vi "ByViServerInterfaceTemplate_CreateClass.vi"(1 "ProjectTreePosition(String or Project Item Ref)":variant, 2 "CreateClassData":T1, 3 "ClassTemplateFolder":path, 5 "error in (no error)":errorcluster, 6 "KeepLvClassRefOpen(False)":bool, 7 "HeaderToApply (take from VIRef or /use 2D-8bit header, Ignored if not wired)":variant) -> (15 "LVClassLibraryRefnum":refnum<vi>, 16 "TemplateVersionUsed":string, 19 "error out":errorcluster)   [LabVIEW 2020]
uses:
  <resource>/Framework/Providers/Open_GDS/ClassProviders/Provider_BaseClassInterface/CreateClassData.ctl
  <resource>/Framework/Providers/Open_GDS/ClassProviders/Common/LvClass_class/GDSLvCLass_ClassSettingsType.ctl
  <resource>/Framework/Providers/Open_GDS/ClassProviders/Common/LvClass_class/GDSLvClass_PlugIn.ctl
  <resource>/Framework/Providers/Open_GDS/ClassProviders/Common/LvClass_class/GDSLvClass_PlugInTypes.ctl
  <resource>/Framework/Providers/Open_GDS/ClassProviders/Provider_BaseClassInterface/ClassWriter_class/ClassWriter.lvclass
  <resource>/Framework/Providers/Open_GDS/ClassProviders/Provider_EndevoGOOP400/ClassWriterGOOP400_class/ClassWriterGOOP400.lvclass
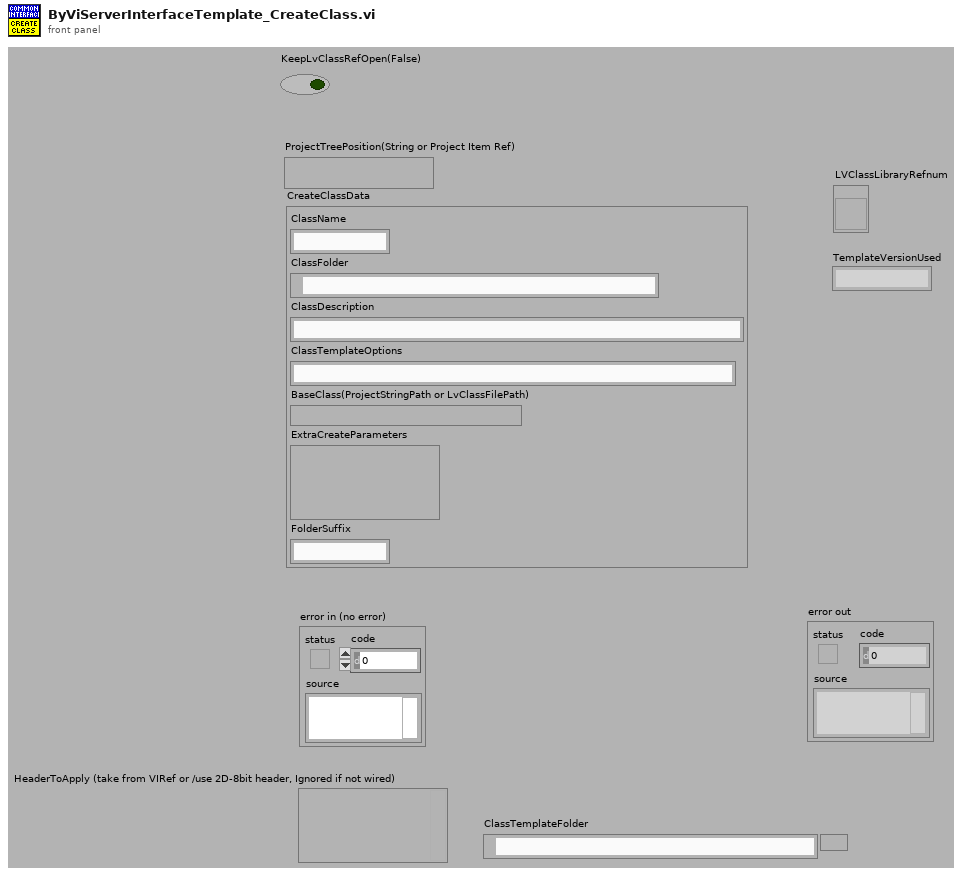
[diagram p1: front panel]
types:
  T1 = typedef "ClassWriter.lvclass/CreateClassData.ctl" = cluster{"ClassName":string, "ClassFolder":path, "ClassDescription":string, "ClassTemplateOptions":string, "BaseClass(ProjectStringPath or LvClassFilePath)":variant, "ExtraCreateParameters":variant, "FolderSuffix":string}
  T2 = cluster{"SubClass":bool, "ClassTemplateFiles":path[], "ClassName":string, "ClassFolder":path, "VIs":refnum<vi>[], "TemplateFolder":path, "ViSubDirs":string[], "TemplateName":string, "BaseClassFolder":path, "RootBaseClassFolder":path, "LvClassPath":path, "ClassRefnum":refnum<vi>, "ProjectRefnum":refnum<vi>, "LvClassFolderPath":path, "BaseClassName":string, "ClassItems":refnum<vi>[], "ViLocked":bool[], "ProjectItemOwner":refnum<vi>, "DeleteFiles":path[], "VIsBefore":refnum<vi>[], "BaseClassPath":path, "BaseConstructorBase":path, "TemplBaseConstructorBase":path, "TemplatePath":path, "TemplateVersion":string, "TemplateParentClass":refnum<vi>, "App":refnum<vi>, "Parent Class":refnum<vi>, "ParentVIs":refnum<vi>[], "TempClass":refnum<vi>}
  T3 = typedef "GDSLvCLass_ClassSettingsType.ctl" = cluster{"ClassProviderName":string, "ClassTemplateUsed":string, "ClassTemplateVersion":string, "ClassDescription":string, "PlugIns":T4[], "ConnectorPanePattern":string}
  T4 = typedef "GDSLvClass_PlugIn.ctl" = cluster{"Type":T5, "ID":string, "Version":string, "Path":path, "Name":string, "Data":variant}
  T5 = typedef "GDSLvClass_PlugInTypes.ctl" = enum16{"DesignPattern", "MethodTypes"}
  T6 = enum32{"invalid lock state", "Not Locked", "Locked (No Password)", "Password-protected"}
  T7 = typedef "Scripting_ConnectorPanePatternType.ctl" = u16
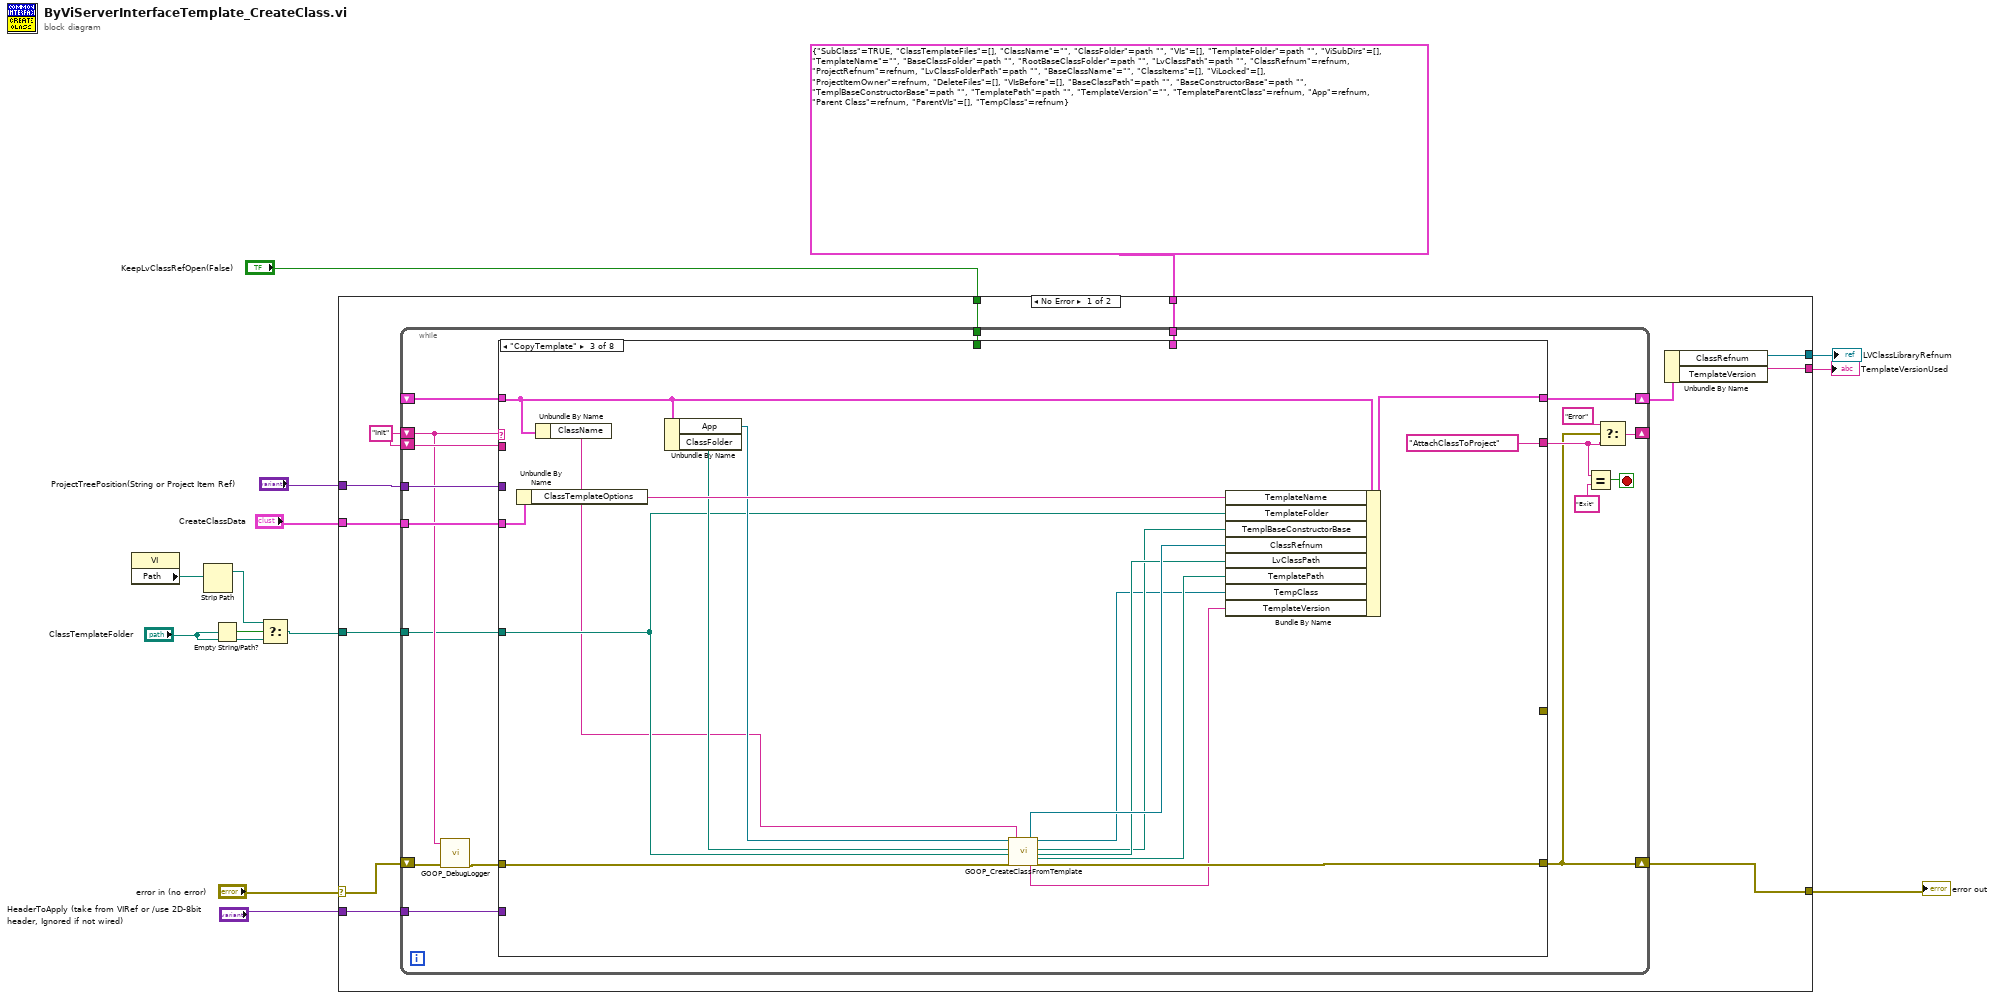
[diagram p0: block diagram]
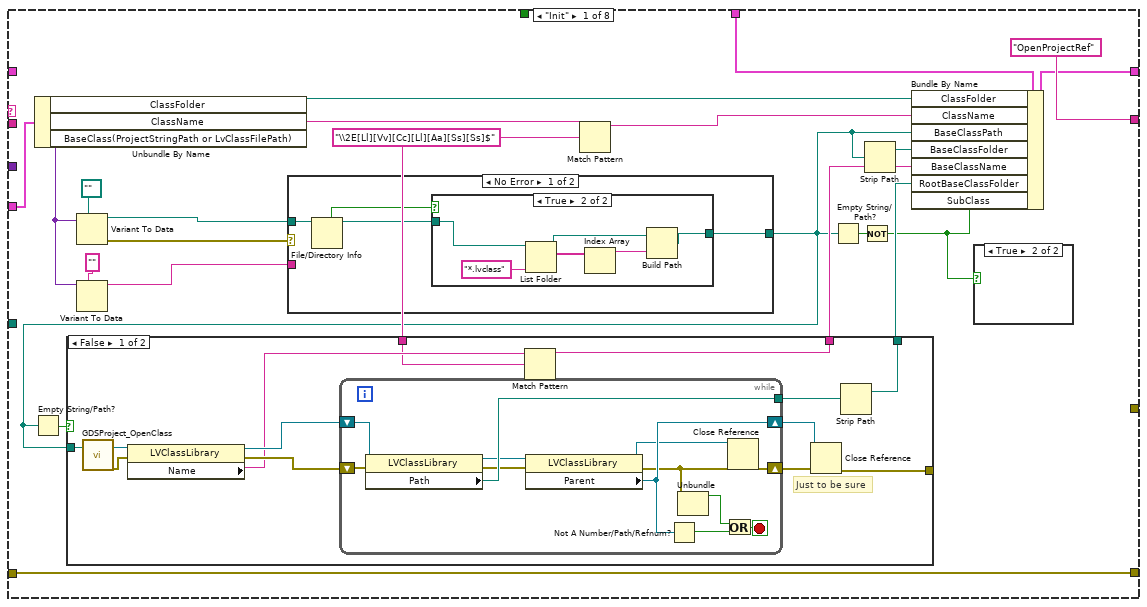
[diagram p2: hidden frame]
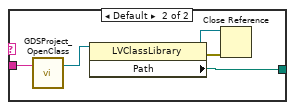
[diagram p7: hidden frame]
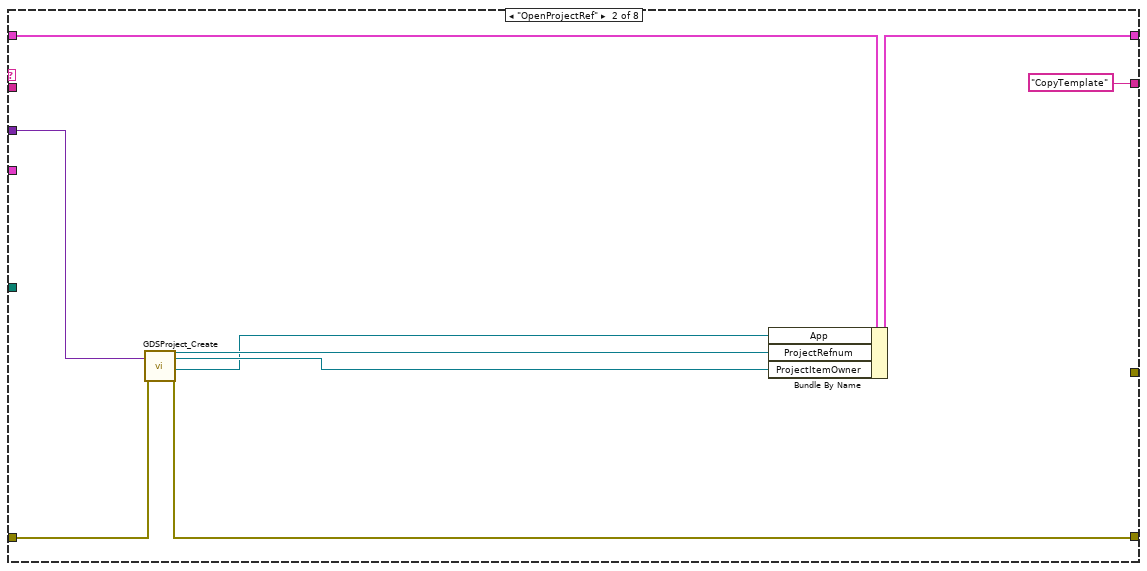
[diagram p8: hidden frame]
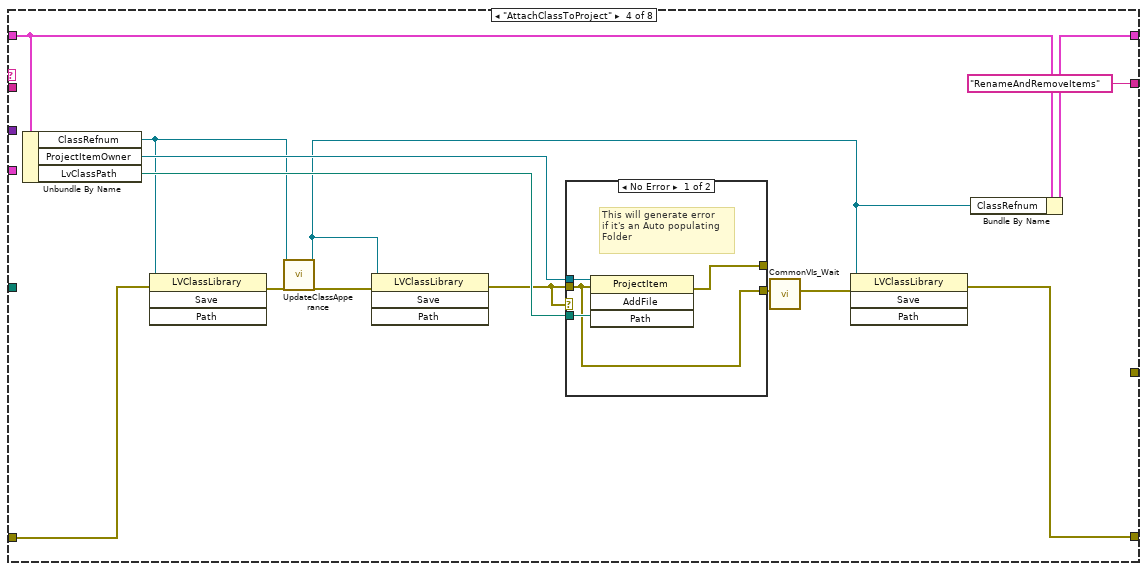
[diagram p9: hidden frame]
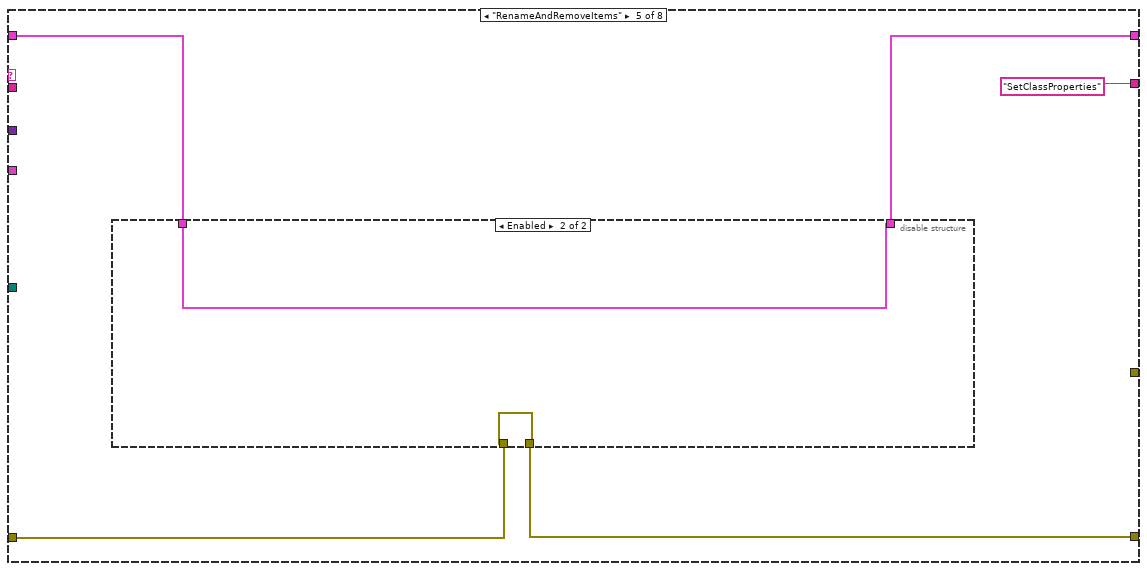
[diagram p11: hidden frame]
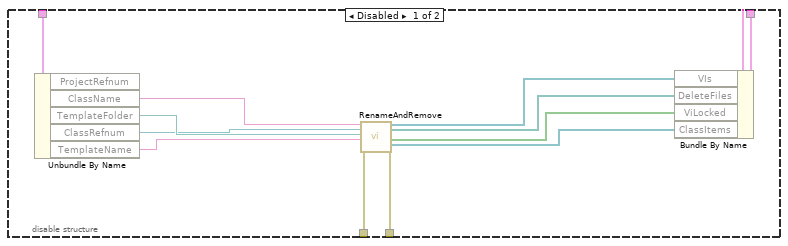
[diagram p12: hidden frame]
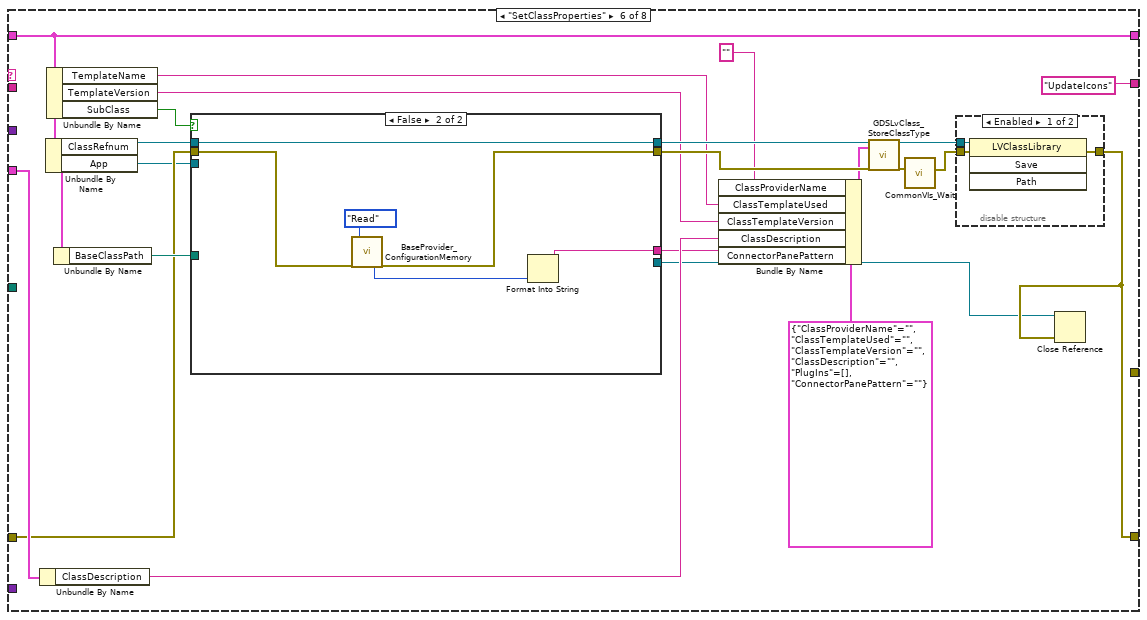
[diagram p13: hidden frame]
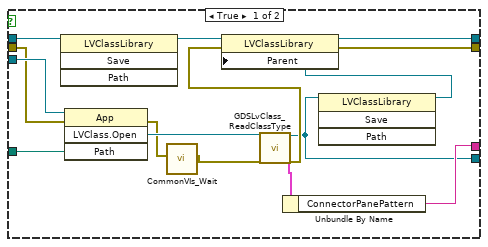
[diagram p15: hidden frame]
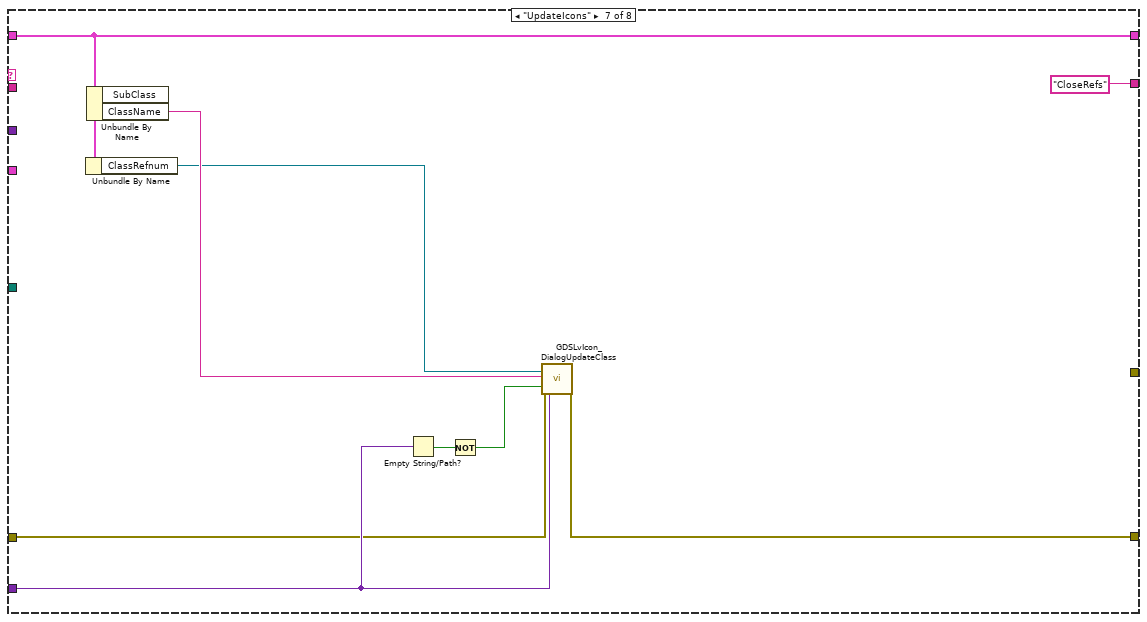
[diagram p16: hidden frame]
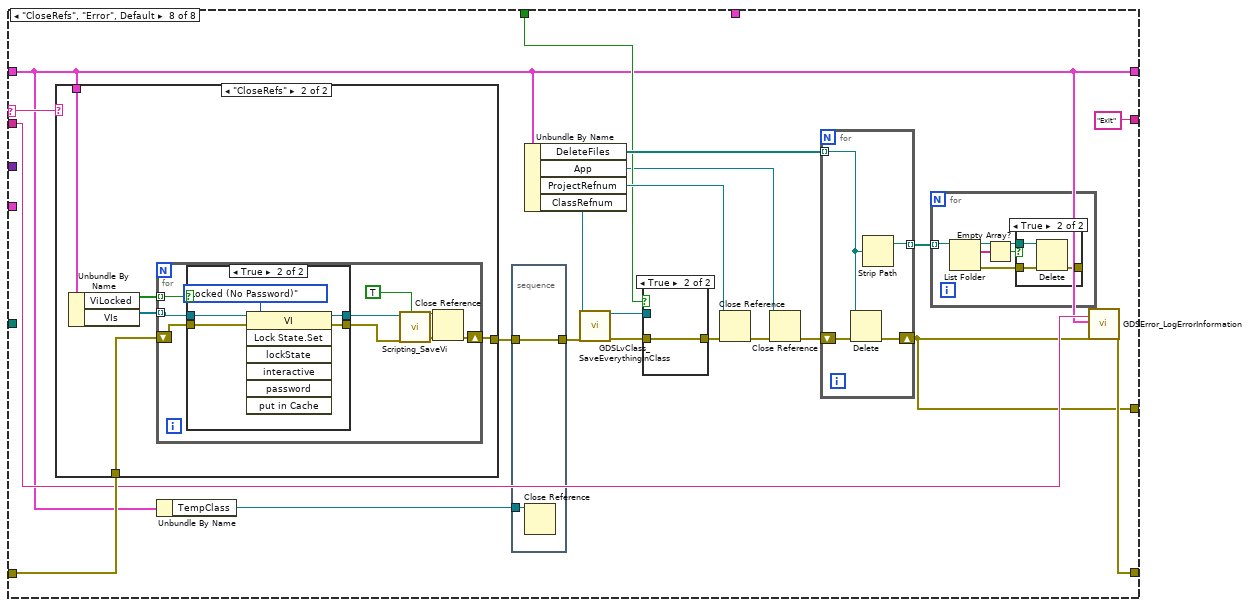
[diagram p17: hidden frame]
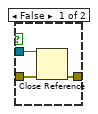
[diagram p18: hidden frame]
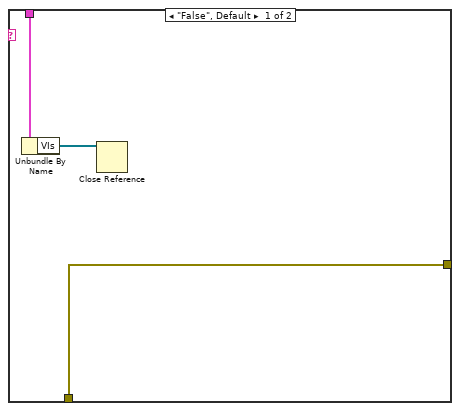
[diagram p20: hidden frame]
diagram:
  n1 = property class="VI"() -> ("Path"=w5:path)  [unwired: 2 in, 2 out]
  n2 = Strip Path(path=w5) -> (stripped path=w2:path)  [unwired: 1 out]
  n3 = Empty String/Path?(string/path="ClassTemplateFolder") -> (empty?=w4:bool)
  n4 = Select(t=w2, s=w4, f="ClassTemplateFolder") -> (s? t:f=w1:path)
  n5 = case shown="No Error" "error in (no error)" {
    selector: "error in (no error)" -> [w17 w292]
    tunnel: [w26 w292] -> w12
    tunnel: "ProjectTreePosition(String or Project Item Ref)" -> [w25 _]
    tunnel: "CreateClassData" -> [w24 _]
    tunnel: "HeaderToApply (take from VIRef or /use 2D-8bit header, Ignored if not wired)" -> [w23 _]
    tunnel: "KeepLvClassRefOpen(False)" -> [w22 _]
    tunnel: [w21 _] -> w7
    tunnel: [w20 _] -> w6
    tunnel: T2 {"SubClass"=TRUE, "ClassTemplateFiles"=[], "ClassName"="", "ClassFolder"=path "", "VIs"=[], "TemplateFolder"=path "", "ViSubDirs"=[], "TemplateName"="", "BaseClassFolder"=path "", "RootBaseClassFolder"=path "", "LvClassPath"=path "", "ClassRefnum"=refnum, "ProjectRefnum"=refnum, "LvClassFolderPath"=path "", "BaseClassName"="", "ClassItems"=[], "ViLocked"=[], "ProjectItemOwner"=refnum, "DeleteFiles"=[], "VIsBefore"=[], "BaseClassPath"=path "", "BaseConstructorBase"=path "", "TemplBaseConstructorBase"=path "", "TemplatePath"=path "", "TemplateVersion"="", "TemplateParentClass"=refnum, "App"=refnum, "Parent Class"=refnum, "ParentVIs"=[], "TempClass"=refnum} ("output cluster") -> [w19 _]
    tunnel: w1 -> [w15 _]
    frame No Error {
      w16 = "Init" ("t")
      n6 = while {
        shift-right: [w36] -> w26
        shift-left: w17 -> [w30]
        shift-right: [w40] -> _
        shift-left: w16 -> [w28]
        shift-right: [w43] -> w18
        shift-left: _ -> [w44]
        tunnel: w19 -> [w38]
        tunnel: w25 -> [w35]
        tunnel: w24 -> [w34]
        shift-left: w16 -> [w33]
        tunnel: w23 -> [w32]
        tunnel: w22 -> [w31]
        tunnel: w15 -> [w27]
        stop <- w41 stop-if-true
        n7 = call <resource>:"GOOP_DebugLogger.vi"("error in (no error)"=w30, "State"=w28) -> ("error out"=w29:errorcluster)  [unwired: 7 in, 2 out]
        n8 = case shown="\"CopyTemplate\"" w28 {
          selector: w28 -> [_ _ _ _ _ _ _ w247]
          tunnel: w44 -> [_ w116 w132 w147 w157 w183 w227 w231]
          tunnel: [w63 w115 w134 w146 w158 w183 w227 w231] -> w43
          tunnel: w29 -> [w66 w114 w126 w141 w155 w184 w221 w248]
          tunnel: [w66 w112 w124 w137 w156 w175 w222 w244] -> w36
          tunnel: ["OpenProjectRef" "CopyTemplate" "AttachClassToProject" "RenameAndRemoveItems" "SetClassProperties" "UpdateIcons" "CloseRefs" "Exit"] -> w37
          tunnel: w38 -> [w59 _ _ _ _ _ _ _]
          tunnel: w35 -> [_ w113 _ _ _ _ _ _]
          tunnel: w34 -> [w58 _ w131 _ _ w190 _ _]
          tunnel: w33 -> [_ _ _ _ _ _ _ w243]
          tunnel: w32 -> [_ _ _ _ _ _ w225 _]
          tunnel: w31 -> [_ _ _ _ _ _ _ w239]
          tunnel: [_ _ _ _ _ _ _ w237] -> _
          tunnel: w27 -> [_ _ w127 _ _ _ _ _]
          frame "Init" {
            w55 = "\\2E[Ll][Vv][Cc][Ll][Aa][Ss][Ss]$" ("regular expression")
            n9 = Unbundle By Name(w58) -> ("ClassFolder"=w52:path, "ClassName"=w51:string, "BaseClass(ProjectStringPath or LvClassFilePath)"=w57:variant)
            n10 = Variant To Data(type=path "" ("path"), Variant=w57) -> (data=w48:path, error out=w49:errorcluster)  [unwired: 1 in]
            n11 = Variant To Data(type="" ("regular expression"), Variant=w57) -> (data=w60:string)  [unwired: 1 in, 1 out]
            n12 = case shown="No Error" w49 {
              tunnel: [w94 w102] -> w46
              tunnel: w60 -> [_ w103]
              tunnel: w48 -> [w93 _]
              frame No Error {
                n13 = File/Directory Info(path=w93) -> (path out=w91:path, directory=w92:bool)  [unwired: 1 in, 5 out]
                n14 = case shown="True" w92 {
                  tunnel: [w95 w97] -> w94
                  tunnel: w91 -> [w95 w96]
                  frame False {
                  }
                  frame True {
                    n15 = List Folder(path=w96, pattern="*.lvclass") -> (path out=w98:path, filenames=w100:string[])  [unwired: 2 in, 2 out]
                    n16 = Index Array(array=w100) -> (element=w99:string)  [unwired: 1 in]
                    n17 = Build Path(base path=w98, name or relative path=w99) -> (appended path=w97:path)
                  }
                }
              }
              frame Error {
                n18 = case shown="\"\"" w103 {
                  tunnel: w103 -> [_ w108]
                  tunnel: [_ w104] -> w102
                  frame "" {
                  }
                  frame Default {
                    n19 = call <resource>:"GDSProject_OpenClass.vi"("ClassPath(FilePath/ProjectTreePath/LvCLassRef)"=w108) -> ("LVClass.Open"=w107:refnum<vi>)  [unwired: 16 in, 2 out]
                    n20 = property class="LVClassLibrary"(reference=w107) -> (reference out=w105:refnum<vi>, error out=w106:errorcluster, "Path"=w104:path)  [unwired: 1 in]
                    n21 = Close Reference(reference=w105, error in (no error)=w106) -> ()  [unwired: 1 out]
                  }
                }
              }
            }
            n22 = Empty String/Path?(string/path=w46) -> (empty?=w53:bool)
            n23 = case shown="False" w53 {
              tunnel: [w76 _] -> w56
              tunnel: w55 -> [w70 _]
              tunnel: [w69 _] -> w54
              tunnel: w46 -> [w68 _]
              tunnel: [w67 _] -> _
              frame False {
                # "Just to be sure"
                n24 = call <resource>:"GDSProject_OpenClass.vi"("ClassPath(FilePath/ProjectTreePath/LvCLassRef)"=w68) -> ("LVClass.Open"=w73:refnum<vi>, "error out"=w75:errorcluster)  [unwired: 16 in, 1 out]
                n25 = property class="LVClassLibrary"(reference=w73, error in=w75) -> (reference out=w72:refnum<vi>, error out=w74:errorcluster, "Name"=w71:string)
                n26 = while {
                  shift-right: [w87] -> w79
                  shift-left: w74 -> [w82]
                  shift-right: [w88] -> w78
                  shift-left: w72 -> [w90]
                  tunnel: [w89] -> w77
                  stop <- w84 stop-if-true
                  n27 = property class="LVClassLibrary"(reference=w90, error in=w82) -> (reference out=w80:refnum<vi>, error out=w81:errorcluster, "Path"=w89:path)
                  n28 = property class="LVClassLibrary"(reference=w80, error in=w81) -> (reference out=w83:refnum<vi>, error out=w87:errorcluster, "Parent"=w88:refnum<vi>)
                  n29 = Not A Number/Path/Refnum?(number/path/refnum=w88) -> (NaN/Path/Refnum?=w85:bool)
                  n30 = Unbundle(w87) -> ("status"=w86:bool)  [unwired: 2 out]
                  n31 = Or(x=w86, y=w85) -> (x .or. y?=w84:bool)
                  n32 = Close Reference(reference=w83) -> ()  [unwired: 1 in, 1 out]
                }
                n33 = Match Pattern(string=w71, regular expression=w70) -> (before substring=w69:string)  [unwired: 1 in, 3 out]
                n34 = Close Reference(reference=w78, error in (no error)=w79) -> (error out=w67:errorcluster)
                n35 = Strip Path(path=w77) -> (stripped path=w76:path)  [unwired: 1 out]
              }
              frame True {
              }
            }
            n36 = Match Pattern(string=w51, regular expression=w55) -> (before substring=w64:string)  [unwired: 1 in, 3 out]
            n37 = Empty String/Path?(string/path=w46) -> (empty?=w47:bool)
            n38 = Not(x=w47) -> (.not. x?=w45:bool)
            n39 = Strip Path(path=w46) -> (stripped path=w50:path)  [unwired: 1 out]
            n40 = Bundle By Name(cluster=w59, "ClassFolder"=w52, "ClassName"=w64, "BaseClassPath"=w46, "BaseClassFolder"=w50, "BaseClassName"=w54, "RootBaseClassFolder"=w56, "SubClass"=w45) -> (w63:T2)
            n41 = case shown="True" w45 {
              frame False {
              }
              frame True {
              }
            }
          }
          frame "OpenProjectRef" {
            n42 = call <resource>:"GDSProject_Create.vi"("ProjectTreePosition(String or Project Item Ref)"=w113, "error in (no error)"=w114) -> ("Project Refnum"=w110:refnum<vi>, "Project Item"=w111:refnum<vi>, "App"=w109:refnum<vi>, "error out"=w112:errorcluster)  [unwired: 14 in]
            n43 = Bundle By Name(cluster=w116, "App"=w109, "ProjectRefnum"=w110, "ProjectItemOwner"=w111) -> (w115:T2)
          }
          frame "CopyTemplate" {
            n44 = Unbundle By Name(w131) -> ("ClassTemplateOptions"=w130:string)
            n45 = Unbundle By Name(w132) -> ("ClassName"=w125:string)
            n46 = Unbundle By Name(w132) -> ("App"=w129:refnum<vi>, "ClassFolder"=w128:path)
            n47 = call <resource>:"GOOP_CreateClassFromTemplate.vi"("Application in"=w129, "ClassFolder"=w128, "TeplateClassFolder"=w127, "error in (no error)"=w126, "ClassName"=w125) -> ("NewClassRef"=w121:refnum<vi>, "TemplateClassVersionString"=w123:string, "TemplateClassRef"=w118:refnum<vi>, "TemplateClassConstructorPath(*Create, *Init)"=w119:path, "NewClassPath"=w120:path, "TemplateClassPath"=w122:path, "error out"=w124:errorcluster)  [unwired: 7 in, 1 out]
            n48 = Bundle By Name(cluster=w132, "TemplateName"=w130, "TemplateFolder"=w127, "TemplBaseConstructorBase"=w119, "ClassRefnum"=w121, "LvClassPath"=w120, "TemplatePath"=w122, "TempClass"=w118, "TemplateVersion"=w123) -> (w134:T2)
          }
          frame "AttachClassToProject" {
            n49 = Unbundle By Name(w147) -> ("ClassRefnum"=w140:refnum<vi>, "ProjectItemOwner"=w148:refnum<vi>, "LvClassPath"=w144:path)
            n50 = invoke class="LVClassLibrary" method="Save"(reference=w140, error in=w141) -> (error out=w142:errorcluster)  [unwired: 2 in, 3 out]
            n51 = call <resource>:"UpdateClassApperance.vi"("ClassRefIn"=w140, "error in (no error)"=w142) -> ("ClassRefOut"=w135:refnum<vi>, "error out"=w139:errorcluster)  [unwired: 16 in]
            n52 = invoke class="LVClassLibrary" method="Save"(reference=w135, error in=w139) -> (error out=w136:errorcluster)  [unwired: 2 in, 3 out]
            n53 = case shown="No Error" w136 {
              tunnel: w148 -> [w152 _]
              tunnel: w144 -> [w151 _]
              tunnel: [w150 w153] -> w143
              tunnel: w136 -> [w150 w153]
              tunnel: [w149 _] -> _
              frame No Error {
                # "This will generate error\nif it's an Auto populating\nFolder"
                n54 = invoke class="ProjectItem" method="AddFile"(reference=w152, error in=w150, "Path"=w151) -> (error out=w149:errorcluster)  [unwired: 1 in, 3 out]
              }
              frame Error {
              }
            }
            n55 = call <resource>:"CommonVIs_Wait.vi"("error in"=w143) -> ("error out"=w138:errorcluster)  [unwired: 9 in]
            n56 = invoke class="LVClassLibrary" method="Save"(reference=w135, error in=w138) -> (error out=w137:errorcluster)  [unwired: 2 in, 3 out]
            n57 = Bundle By Name(cluster=w147, "ClassRefnum"=w135) -> (w146:T2)
          }
          frame "RenameAndRemoveItems" {
            n58 = disable-structure shown="Enabled" {
              disable-tunnel: [w168 w171] -> w158
              disable-tunnel: w157 -> [w166 w171]
              disable-tunnel: [w164 w172] -> w156
              disable-tunnel: w155 -> [w163 w172]
              frame Disabled {
                n59 = Unbundle By Name(w166) -> ("ClassName"=w170:string, "TemplateFolder"=w167:path, "ClassRefnum"=w165:refnum<vi>, "TemplateName"=w159:string)  [unwired: 1 out]
                n60 = call <resource>:"RenameAndRemove.vi"("ClassName"=w170, "ClassRefnum"=w165, "TemplateFolder"=w167, "TemplateName"=w159, "error in"=w163) -> ("ViRefsOut"=w169:refnum<vi>[], "DeleteFiles"=w162:path[], "ItemLocked"=w161:bool[], "Items"=w160:refnum<vi>[], "error out"=w164:errorcluster)  [unwired: 10 in]
                n61 = Bundle By Name(cluster=w166, "VIs"=w169, "DeleteFiles"=w162, "ViLocked"=w161, "ClassItems"=w160) -> (w168:T2)
              }
              frame Enabled {
              }
            }
          }
          frame "SetClassProperties" {
            n62 = Unbundle By Name(w190) -> ("ClassDescription"=w187:string)
            n63 = Unbundle By Name(w183) -> ("ClassRefnum"=w185:refnum<vi>, "App"=w180:refnum<vi>)
            n64 = Unbundle By Name(w183) -> ("TemplateName"=w186:string, "TemplateVersion"=w181:string, "SubClass"=w194:bool)
            n65 = Unbundle By Name(w183) -> ("BaseClassPath"=w193:path)
            n66 = case shown="False" w194 {
              tunnel: w185 -> [w202 w219]
              tunnel: [w213 w219] -> w192
              tunnel: w184 -> [w206 w215]
              tunnel: [w212 w214] -> w191
              tunnel: w193 -> [w211 _]
              tunnel: w180 -> [w207 _]
              tunnel: [w208 w216] -> w179
              tunnel: [w200 _] -> w174
              frame True {
                n67 = invoke class="LVClassLibrary" method="Save"(reference=w202) -> (reference out=w201:refnum<vi>)  [unwired: 3 in, 3 out]
                n68 = invoke class="App" method="LVClass.Open"(reference=w207, error in=w206, "Path"=w211) -> (error out=w205:errorcluster, "LVClass.Open"=w210:refnum<vi>)  [unwired: 1 in, 2 out]
                n69 = call <resource>:"CommonVIs_Wait.vi"("error in"=w205) -> ("error out"=w204:errorcluster)  [unwired: 9 in]
                n70 = call <resource>:"GDSLvClass_ReadClassType.vi"("Class Refnum In"=w210, "error in (no error)"=w204) -> ("Class Refnum Out"=w200:refnum<vi>, "ClassSettings"=w209:T3, "error out"=w203:errorcluster)  [unwired: 15 in]
                n71 = Unbundle By Name(w209) -> ("ConnectorPanePattern"=w208:string)
                n72 = invoke class="LVClassLibrary" method="Save"(reference=w200) -> (reference out=w199:refnum<vi>)  [unwired: 3 in, 3 out]
                n73 = property class="LVClassLibrary"(reference=w201, error in=w203, "Parent"=w199) -> (reference out=w213:refnum<vi>, error out=w212:errorcluster)
              }
              frame False {
                n74 = call <resource>:"BaseProvider_ConfigurationMemory.vi"("error in (no error)"=w215, "Action"=enum16{"Read", "Load", "Save"}."Read") -> ("PatternOut"=w218:T7, "error out"=w214:errorcluster)  [unwired: 11 in, 5 out]
                n75 = Format Into String(w218) -> (resulting string=w216:string)  [unwired: 3 in, 1 out]
              }
            }
            n76 = Bundle By Name(cluster=T3 {"ClassProviderName"="", "ClassTemplateUsed"="", "ClassTemplateVersion"="", "ClassDescription"="", "PlugIns"=[], "ConnectorPanePattern"=""} ("ClassSettings"), "ClassProviderName"="", "ClassTemplateUsed"=w186, "ClassTemplateVersion"=w181, "ClassDescription"=w187, "ConnectorPanePattern"=w179) -> (w188:T3)
            n77 = call <resource>:"GDSLvClass_StoreClassType.vi"("Class Refnum In"=w192, "ClassSettings"=w188, "error in (no error)"=w191) -> ("Class Refnum Out"=w178:refnum<vi>, "error out"=w177:errorcluster)  [unwired: 15 in]
            n78 = call <resource>:"CommonVIs_Wait.vi"("error in"=w177) -> ("error out"=w176:errorcluster)  [unwired: 9 in]
            n79 = disable-structure shown="Enabled" {
              disable-tunnel: [w197 w198] -> w175
              disable-tunnel: w178 -> [w196 _]
              disable-tunnel: w176 -> [w195 w198]
              frame Enabled {
                n80 = invoke class="LVClassLibrary" method="Save"(reference=w196, error in=w195) -> (error out=w197:errorcluster)  [unwired: 2 in, 3 out]
              }
              frame Disabled {
              }
            }
            n81 = Close Reference(reference=w174, error in (no error)=w175) -> ()  [unwired: 1 out]
          }
          frame "UpdateIcons" {
            n82 = Unbundle By Name(w227) -> ("ClassRefnum"=w226:refnum<vi>)
            n83 = Unbundle By Name(w227) -> ("ClassName"=w228:string)  [unwired: 1 out]
            n84 = Empty String/Path?(string/path=w225) -> (empty?=w224:bool)
            n85 = Not(x=w224) -> (.not. x?=w223:bool)
            n86 = call <resource>:"GDSLvIcon_DialogUpdateClass.vi"("ClassPath(FilePath/ProjectTreePath/LvCLassRef)"=w226, "ClassName"=w228, "AutoUpdate"=w223, "error in (no error)"=w221, "HeaderToApply (take from VIRef or /use 2D-8bit header, Ignored if not wired)"=w225) -> ("error out"=w222:errorcluster)  [unwired: 11 in, 3 out]
          }
          frame "CloseRefs", "Error", Default {
            n87 = case shown="\"CloseRefs\"" w247 {
              tunnel: w248 -> [w270 w274]
              tunnel: w231 -> [w269 w273]
              tunnel: [w270 w272] -> w232
              frame "False", Default {
                n88 = Unbundle By Name(w269) -> ("VIs"=w268:refnum<vi>[])
                n89 = Close Reference(reference=w268) -> ()  [unwired: 1 in, 1 out]
              }
              frame "CloseRefs" {
                n90 = Unbundle By Name(w273) -> ("ViLocked"=w271:bool[], "VIs"=w275:refnum<vi>[])
                n91 = for {
                  tunnel: w275 -> [w280] mode=indexing
                  shift-right: [w276] -> w272
                  shift-left: w274 -> [w281]
                  tunnel: w271 -> [w277] mode=indexing
                  n92 = case shown="True" w277 {
                    tunnel: w281 -> [w285 w291]
                    tunnel: w280 -> [w286 w290]
                    tunnel: [w285 w289] -> w279
                    tunnel: [w286 w288] -> w278
                    frame False {
                    }
                    frame True {
                      n93 = invoke class="VI" method="Lock State.Set"(reference=w290, error in=w291, "lockState"=T6."Locked (No Password)" ("Lock State")) -> (reference out=w288:refnum<vi>, error out=w289:errorcluster)  [unwired: 4 in, 5 out]
                    }
                  }
                  n94 = call <resource>:"Scripting_SaveVi.vi"("ForceResaving(False)"=TRUE, "error in (no error)"=w279, "VIRefToSaveIn"=w278) -> ("error out"=w284:errorcluster, "VIRefToSaveOut"=w283:refnum<vi>)  [unwired: 7 in]
                  n95 = Close Reference(reference=w283, error in (no error)=w284) -> (error out=w276:errorcluster)
                }
              }
            }
            n96 = Unbundle By Name(w231) -> ("TempClass"=w230:refnum<vi>)
            n97 = stacked-sequence {
              tunnel: w232 -> [w250]
              tunnel: [w250] -> w229
              tunnel: w230 -> [w251]
              frame #0 {
                n98 = Close Reference(reference=w251) -> ()  [unwired: 1 in, 1 out]
              }
            }
            n99 = Unbundle By Name(w231) -> ("DeleteFiles"=w242:path[], "App"=w234:refnum<vi>, "ProjectRefnum"=w245:refnum<vi>, "ClassRefnum"=w241:refnum<vi>)
            n100 = call <resource>:"GDSLvClass_SaveEverythingInClass.vi"("ClassRefIn"=w241, "error in"=w229) -> ("ClassRefOut"=w236:refnum<vi>, "error out"=w238:errorcluster)  [unwired: 16 in]
            n101 = case shown="True" w239 {
              tunnel: [w254 w255] -> w246
              tunnel: w238 -> [w253 w255]
              tunnel: w236 -> [w252 _]
              frame False {
                n102 = Close Reference(reference=w252, error in (no error)=w253) -> (error out=w254:errorcluster)
              }
              frame True {
              }
            }
            n103 = Close Reference(reference=w245, error in (no error)=w246) -> (error out=w235:errorcluster)
            n104 = Close Reference(reference=w234, error in (no error)=w235) -> (error out=w233:errorcluster)
            n105 = for {
              shift-right: [w266] -> w237
              shift-left: w233 -> [w267]
              tunnel: w242 -> [w265] mode=indexing
              tunnel: [w264] -> w240 mode=indexing
              n106 = Delete(path (use dialog)=w265, error in=w267) -> (error out=w266:errorcluster)  [unwired: 3 in, 2 out]
              n107 = Strip Path(path=w265) -> (stripped path=w264:path)  [unwired: 1 out]
            }
            n108 = for {
              tunnel: w240 -> [w260] mode=indexing
              n109 = List Folder(path=w260) -> (path out=w256:path, filenames=w259:string[], error out=w257:errorcluster)  [unwired: 3 in, 1 out]
              n110 = Empty Array?(array=w259) -> (empty?=w258:bool)
              n111 = case shown="True" w258 {
                tunnel: w257 -> [_ w263]
                tunnel: w256 -> [_ w262]
                tunnel: [_ w261] -> _
                frame False {
                }
                frame True {
                  n112 = Delete(path (use dialog)=w262, error in=w263) -> (error out=w261:errorcluster)  [unwired: 3 in, 2 out]
                }
              }
            }
            n113 = call <resource>:"GDSError_LogErrorInformation.vi"("State"=w243, "LocalVariableData"=w231, "error in (no error)"=w237) -> ("error out"=w244:errorcluster)  [unwired: 16 in]
          }
        }
        n114 = Equal?(x=w37, y="Exit") -> (x = y?=w41:bool)
        n115 = Select(t="Error", s=w36, f=w37) -> (s? t:f=w40:string)
      }
      n116 = Unbundle By Name(w18) -> ("ClassRefnum"=w21:refnum<vi>, "TemplateVersion"=w20:string)
    }
    frame Error {
    }
  }
  "error out" <- w12
  "LVClassLibraryRefnum" <- w7
  "TemplateVersionUsed" <- w6
